vi "CRYView Pic  Command Get.vi"() -> (0 "nData_Out":i32, 2 "cCommand_Out":T1)   [LabVIEW 2013]
uses:
  CRYView Global.vi
panel:
  out "Start_Positin 2":T2
  in  "ToolBar Click":bool
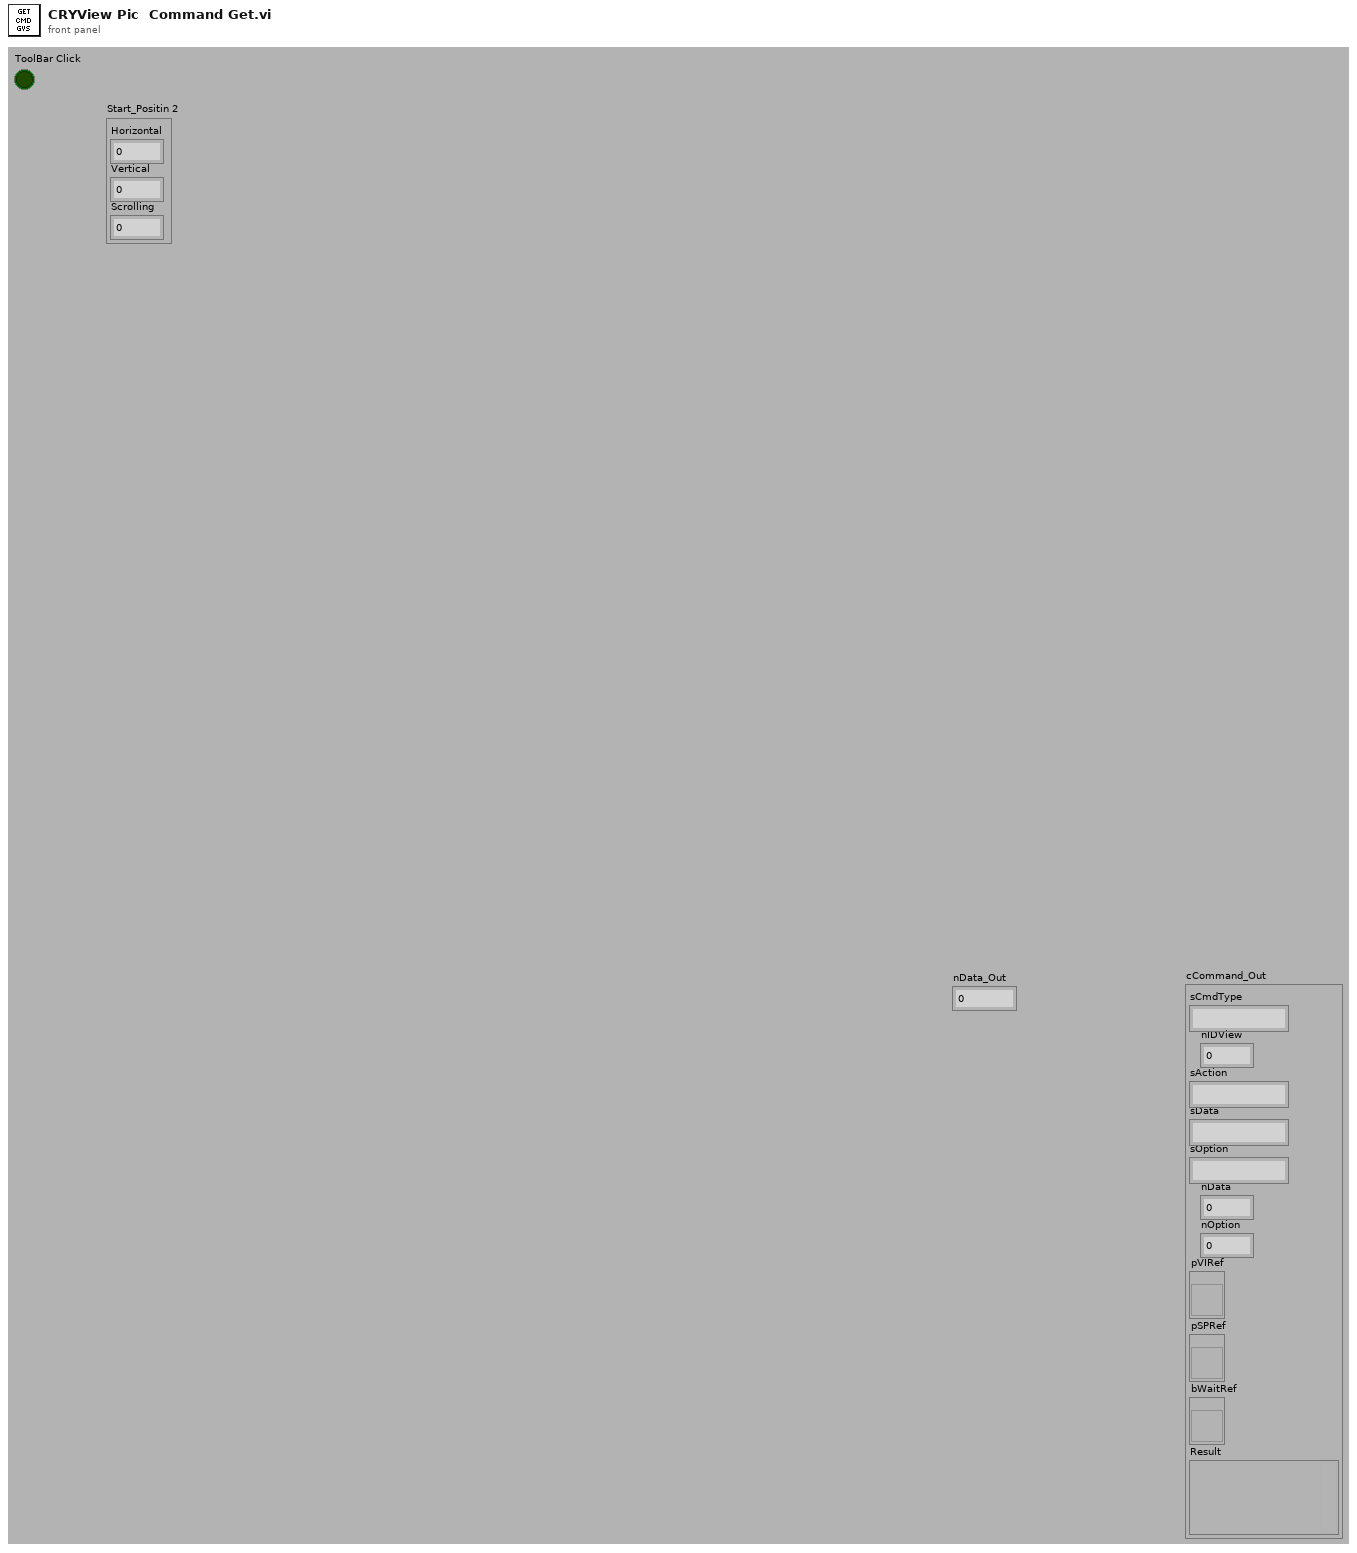
[diagram p1: front panel]
types:
  T1 = cluster{"sCmdType":string, "nIDView":i32, "sAction":string, "sData":string, "sOption":string, "nData":i32, "nOption":i32, "pVIRef":refnum<vi>, "pSPRef":refnum<vi>, "bWaitRef":refnum<vi>, "Result":variant}
  T2 = cluster{"Horizontal":i32, "Vertical":i32, "Scrolling":i32}
  T3 = cluster{"sCmdType":string, "nIDView":i32, "sAction":string, "sData":string, "sOption":string, "nData":i32, "nOption":i32, "pVIRef":refnum<vi>, "pSPRef":refnum<vi>, "bWaitRef":refnum<vi>, "Result":variant}[]
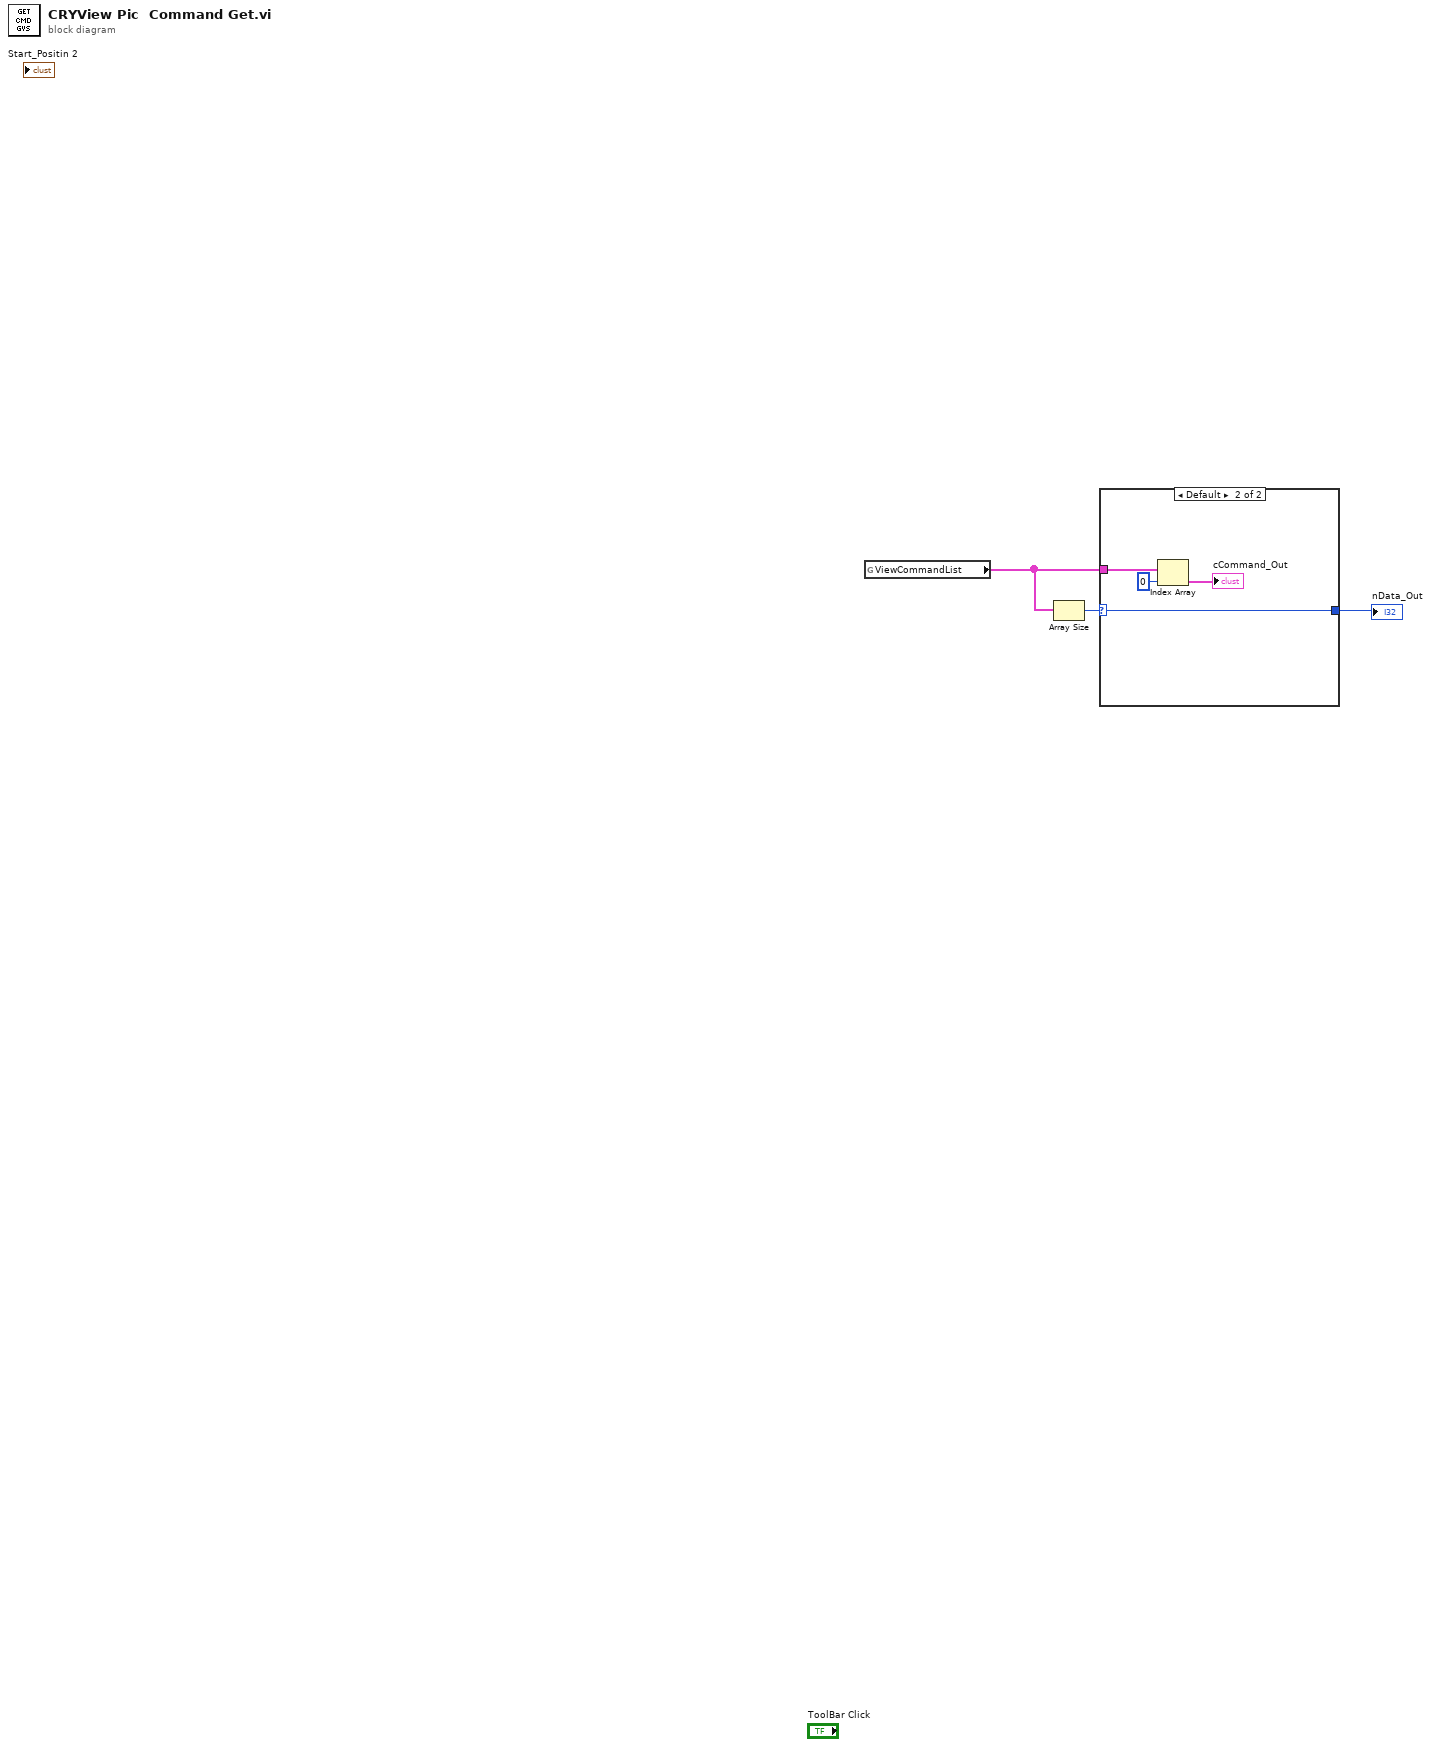
[diagram p0: block diagram]
diagram:
  n1 = global read "CRYView Global.vi" "ViewCommandList"() -> (w2:T3)
  n2 = Array Size(array=w2) -> (size(s)=w3:i32)
  n3 = case shown="Default" w3 {
    selector: w3 -> [w4 w5]
    tunnel: w2 -> [_ w7]
    tunnel: [w4 w5] -> w1
    frame 0 {
    }
    frame Default {
      n4 = Index Array(array=w7, index=0) -> (element=→"cCommand_Out":T1)
    }
  }
  "nData_Out" <- w1
